vi "Get Run Parameters.vi"(8 "error in":errorcluster, 11 "TDMS in":refnum<class "TDMS.lvclass">) -> (0 "error out":errorcluster, 1 "run params":variant[](array[variant]), 2 "param names":string[](array[string]), 3 "TDMS out":refnum<class "TDMS.lvclass">)   [LabVIEW 2011, in "TDMS.lvclass"]
uses:
  TDMS.lvclass
  TDMS.lvclass/TDMS.ctl
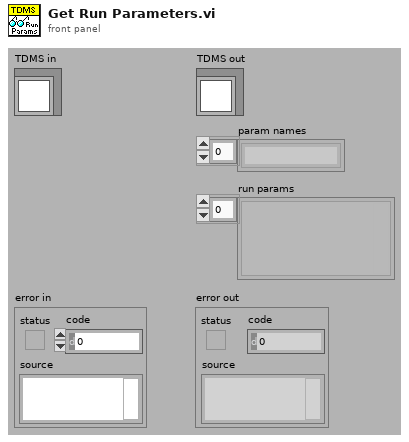
[diagram p1: front panel]
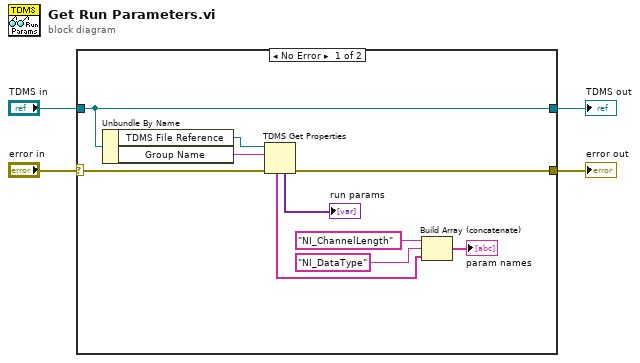
[diagram p0: block diagram]
diagram:
  n1 = case shown="No Error" "error in" {
    selector: "error in" -> [w13 w15]
    tunnel: [w12 w15] -> w1
    tunnel: [w14 w16] -> w2
    tunnel: "TDMS in" -> [w14 w16]
    frame No Error {
      n2 = Unbundle By Name(w14) -> ("TDMS File Reference"=w10:refnum<k34>, "Group Name"=w11:string)
      n3 = TDMS Get Properties(8:w13, 10:w11, 11:w10) -> (0:w12:errorcluster, 4:→"run params":variant[], 6:w6:string[])  [unwired: 3 in, 3 out]
      n4 = Build Array (concatenate)("NI_ChannelLength" ("new element/subarray"), "NI_DataType" ("element"), w6) -> (→"param names":string[])
    }
    frame Error {
    }
  }
  "error out" <- w1
  "TDMS out" <- w2
